vi "Valves and Pumps Initializer.vi"() -> (3 "Devices":T1[](array[typedef]))   [LabVIEW 2011]
uses:
  Valve_Pump.ctl
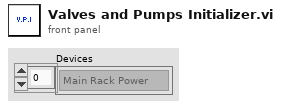
[diagram p1: front panel]
types:
  T1 = typedef "Valve_Pump.ctl" = enum16{"Main Rack Power", "Pump Power", "Valve Power", "V4", "V5", "V6", "V7", "V8", "V9", "V10", "V11", "V12", "V13", "V14", "V15", "V18", "V19", "V20", "V21", "V22", "V23", "V24", "V25", "V26", "V27", "V28", "V29", "V30", "V31", "V32", "V33", "V34", "Pump A", "Pump B", "Pump C", "Pump D"}
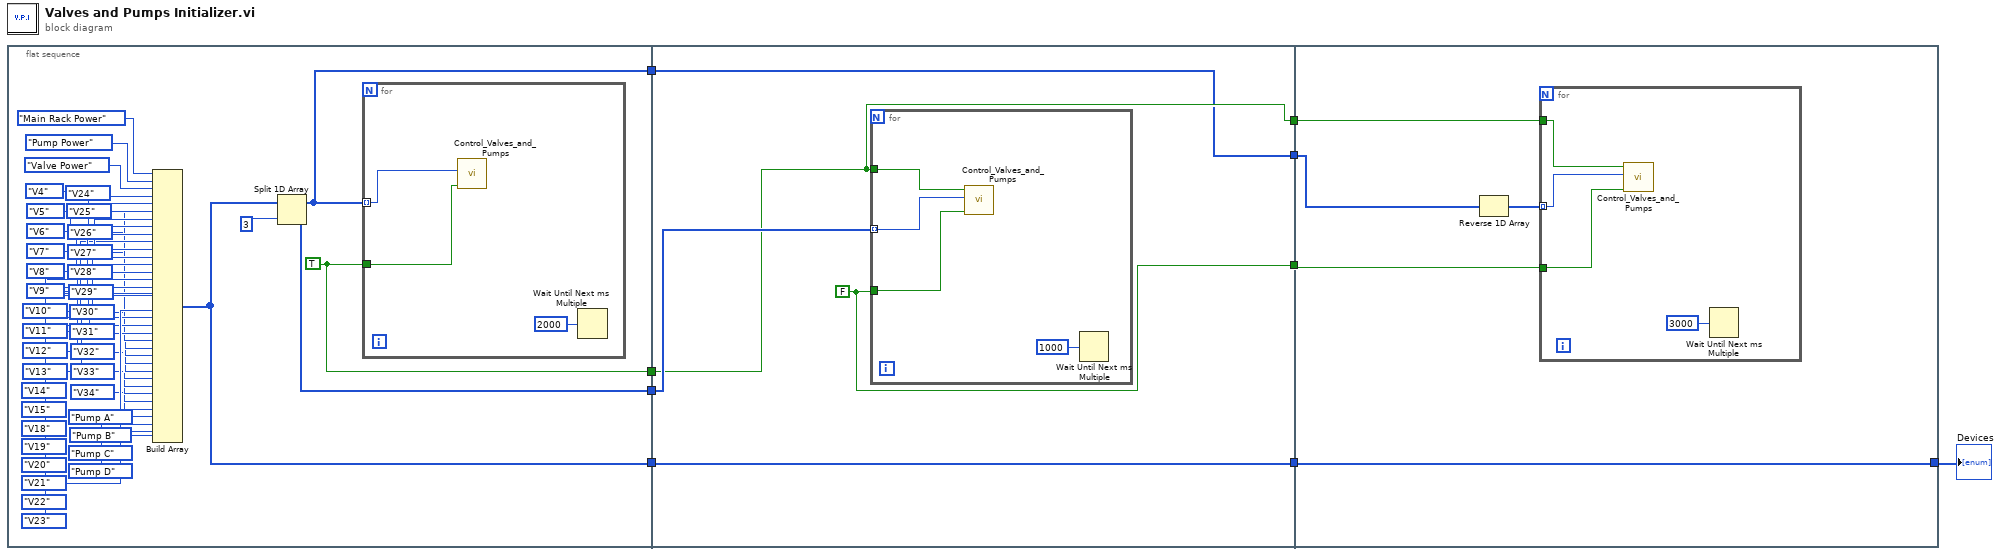
[diagram p0: block diagram]
diagram:
  n1 = flat-sequence {
    tunnel: [w10] -> w8
    tunnel: [w13] -> w7
    tunnel: [w12] -> w6
    tunnel: [w11] -> w5
    tunnel: w8 -> [w55]
    tunnel: [w55] -> w4
    tunnel: w7 -> [w56]
    tunnel: w6 -> [w57]
    tunnel: w5 -> [w54]
    tunnel: [w56] -> w3
    tunnel: [w58] -> w2
    tunnel: [w54] -> w1
    tunnel: [w63] -> w9
    tunnel: w4 -> [w63]
    tunnel: w3 -> [w67]
    tunnel: w2 -> [w64]
    tunnel: w1 -> [w66]
    frame #0 {
      w13 = TRUE
      n2 = Build Array(Valve_Pump."Main Rack Power" ("Device"), Valve_Pump."Pump Power" ("Device"), Valve_Pump."Valve Power" ("Device"), Valve_Pump."V4" ("Device"), Valve_Pump."V5" ("Device"), Valve_Pump."V6" ("Device"), Valve_Pump."V7" ("Device"), Valve_Pump."V8" ("Device"), Valve_Pump."V9" ("Device"), Valve_Pump."V10" ("Device"), Valve_Pump."V11" ("Device"), Valve_Pump."V12" ("Device"), Valve_Pump."V13" ("Device"), Valve_Pump."V14" ("Device"), Valve_Pump."V15" ("Device"), Valve_Pump."V18" ("Device"), Valve_Pump."V19" ("Device"), Valve_Pump."V20" ("Device"), Valve_Pump."V21" ("Device"), Valve_Pump."V22" ("Device"), Valve_Pump."V23" ("Device"), Valve_Pump."V24" ("Device"), Valve_Pump."V25" ("Device"), Valve_Pump."V26" ("Device"), Valve_Pump."V27" ("Device"), Valve_Pump."V28" ("Device"), Valve_Pump."V29" ("Device"), Valve_Pump."V30" ("Device"), Valve_Pump."V31" ("Device"), Valve_Pump."V32" ("Device"), Valve_Pump."V33" ("Device"), Valve_Pump."V34" ("Device"), Valve_Pump."Pump A" ("Device"), Valve_Pump."Pump B" ("Device"), Valve_Pump."Pump C" ("Device"), Valve_Pump."Pump D" ("Device")) -> (w10:T1[])
      n3 = Split 1D Array(array=w10, index=3) -> (first subarray=w11:T1[], second subarray=w12:T1[])
      n4 = for {
        tunnel: w11 -> [w53] mode=indexing
        tunnel: w13 -> [w52]
        n5 = call "Control_Valves_and_Pumps.vi"("Set state:"=w52, "Device"=w53) -> ()  [unwired: 10 in]
        n6 = Wait Until Next ms Multiple(millisecond multiple=2000) -> ()  [unwired: 1 out]
      }
    }
    frame #1 {
      w58 = FALSE
      n7 = for {
        tunnel: w57 -> [w62] mode=indexing
        tunnel: w58 -> [w61]
        tunnel: w56 -> [w60]
        n8 = call "Control_Valves_and_Pumps.vi"("Set state:"=w61, "Device"=w62, "Mode of Operation"=w60) -> ()  [unwired: 9 in]
        n9 = Wait Until Next ms Multiple(millisecond multiple=1000) -> ()  [unwired: 1 out]
      }
    }
    frame #2 {
      n10 = Reverse 1D Array(array=w66) -> (reversed array=w65:T1[])
      n11 = for {
        tunnel: w65 -> [w71] mode=indexing
        tunnel: w64 -> [w70]
        tunnel: w67 -> [w69]
        n12 = call "Control_Valves_and_Pumps.vi"("Set state:"=w70, "Device"=w71, "Mode of Operation"=w69) -> ()  [unwired: 9 in]
        n13 = Wait Until Next ms Multiple(millisecond multiple=3000) -> ()  [unwired: 1 out]
      }
    }
  }
  "Devices" <- w9
